vi "UI Initialize.vi"(8 "error in (no error)":errorcluster, 11 "UI ActorTop in":refnum<class "UI_Left_Right.lvclass">) -> (0 "error out":errorcluster, 3 "UI ActorTop out":refnum<class "UI_Left_Right.lvclass">)   [LabVIEW 2021, in "UI_Left_Right.lvclass"]
doc: "UI: Initialize\n2015-03-18 16:27:22\n蒋松\njiangsong@outlook.com"
uses:
  UI_Left_Right.lvclass
  C:/Program Files (x86)/National Instruments/LabVIEW 2021/user.lib/John_Lib/AbstractActorTemplate/AbstractActorTemplate/UIActorTop.lvclass
  <userlib>/John_Lib/AbstractActorTemplate/AbstractActorTemplate/UIActorTop.lvclass
  UI_Left_Right.lvclass/UI_Left_Right.ctl
  <vilib>/ActorFramework/Actor/Actor.lvclass
  C:/Program Files (x86)/National Instruments/LabVIEW 2021/vi.lib/ActorFramework/Actor/Actor.lvclass
  C:/Program Files (x86)/National Instruments/LabVIEW 2021/project/Create Actor from Template/_UI_Left_Right/UI_Left_Right.lvclass
  C:/Program Files (x86)/National Instruments/LabVIEW 2021/user.lib/John_Lib/Interfaces/InsertLeftSubPanel/InsertLeftSubPanel.lvclass
  C:/Program Files (x86)/National Instruments/LabVIEW 2021/user.lib/John_Lib/Interfaces/InsertRightSubPanel/InsertRightSubPanel.lvclass
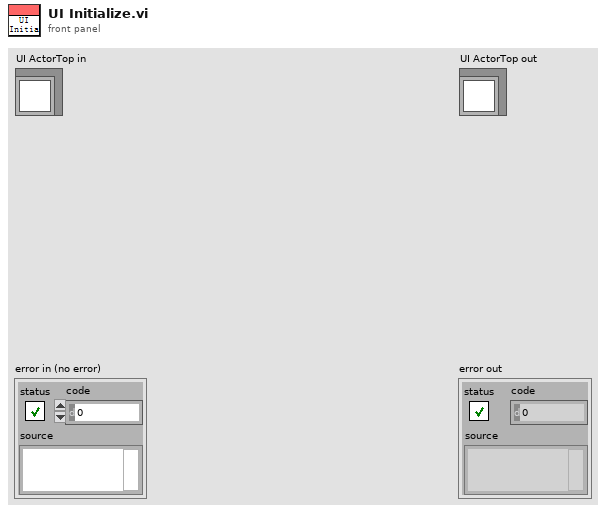
[diagram p1: front panel]
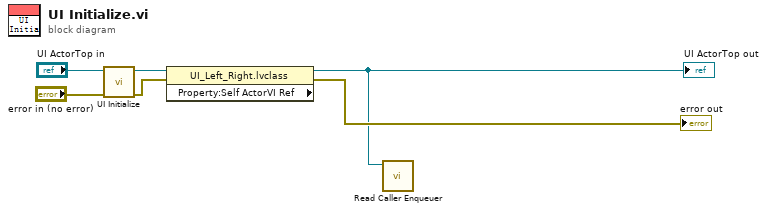
[diagram p0: block diagram]
diagram:
  n1 = call-parent "UI Initialize.vi"("error in (no error)"="error in (no error)", "UI ActorTop in"="UI ActorTop in") -> ("error out"=w3:errorcluster, "UI ActorTop out"=w5:refnum<class "UI_Left_Right.lvclass">)  [unwired: 8 in]
  n2 = property class="UI_Left_Right.lvclass" props=["Property:Self ActorVI Ref"](reference=w5, error in=w3) -> (reference out=w1:refnum<class "UI_Left_Right.lvclass">, error out=→"error out":errorcluster)  [unwired: 1 out]
  "UI ActorTop out" <- w1
  n3 = call <vilib>:"Read Caller Enqueuer.vi"("Actor"=w1) -> ()  [unwired: 10 in, 1 out]
